vi "FT10_Semi-Auto Tester.vi"(7 "Read/ Write":T8, 8 "Error In":errorcluster, 10 "Semi-Auto Cluster in":T1[](array[typedef]), 11 "Path":path=path "FT10_rev2/Semi-Auto Commands.csv") -> (0 "Error Out":errorcluster, 2 "Semi-Auto Cluster out":T1[](array[typedef]), 3 "Semi-Auto 2-D Array out":T7)   [LabVIEW 2015]
uses:
  LV2024/NI Online Practice/CLD Practice/cld_success_package/Preparation_Materials/CLD 6/CLD 6 CSV file enum.ctl
  Controls/Control_Semi-Auto 2-D Array.ctl
  Controls/Control_Semi-Auto Cluster.ctl
  Controls/Control_Semi-Auto Unitherm Load.ctl
  Controls/Control_Semi-Auto Port.ctl
  Controls/Control_Semi-Auto Mode.ctl
  Controls/Control_Semi-Auto Power Level.ctl
  Controls/Control_Semi-Auto Activation Duration.ctl
  Controls/Control_Semi-Auto 1-D Array.ctl
  <vilib>/Utility/file.llb/Read Delimited Spreadsheet (string).vi
  <vilib>/Utility/file.llb/Write Delimited Spreadsheet (string).vi
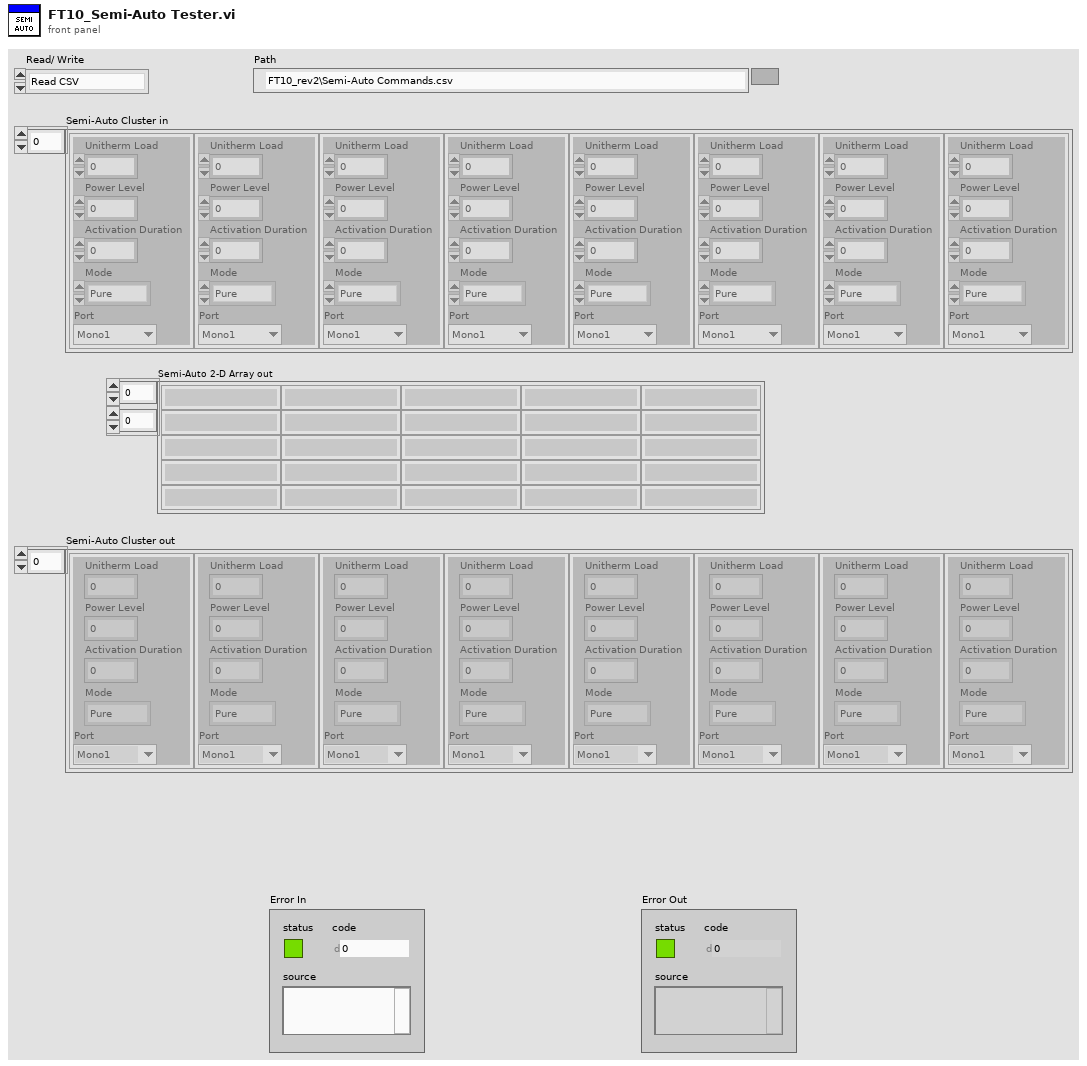
[diagram p1: front panel]
types:
  T1 = typedef "Control_Semi-Auto Cluster.ctl" = cluster{"Unitherm Load":T2, "Port":T3, "Mode":T4, "Power Level":T5, "Activation Duration":T6}
  T2 = typedef "Control_Semi-Auto Unitherm Load.ctl" = i32
  T3 = typedef "Control_Semi-Auto Port.ctl" = enum16{"Mono1", "Mono2", "Bipolar", "Ligasure", "Error"}
  T4 = typedef "Control_Semi-Auto Mode.ctl" = enum16{"Pure", "Blend", "Spray", "Fulgerate", "Standard", "Macro", "Precision", "Ligasure", "Error"}
  T5 = typedef "Control_Semi-Auto Power Level.ctl" = i32
  T6 = typedef "Control_Semi-Auto Activation Duration.ctl" = i32
  T7 = typedef "Control_Semi-Auto 2-D Array.ctl" = string[][]
  T8 = typedef "CLD 6 CSV file enum.ctl" = enum16{"Read CSV", "Write CSV"}
  T9 = typedef "Control_Semi-Auto 1-D Array.ctl" = string[]
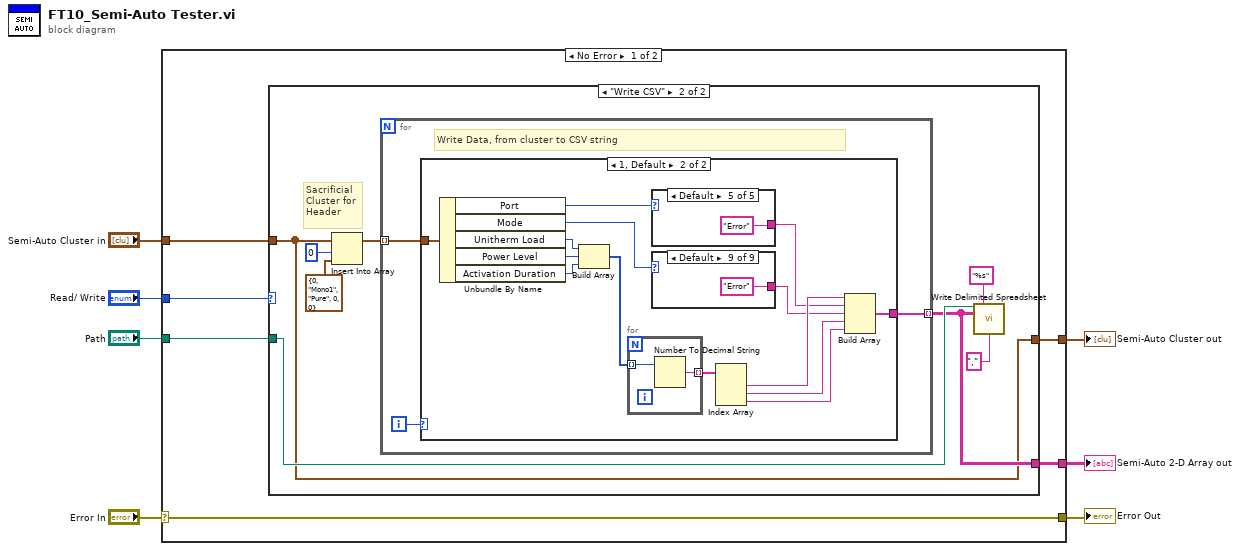
[diagram p0: block diagram]
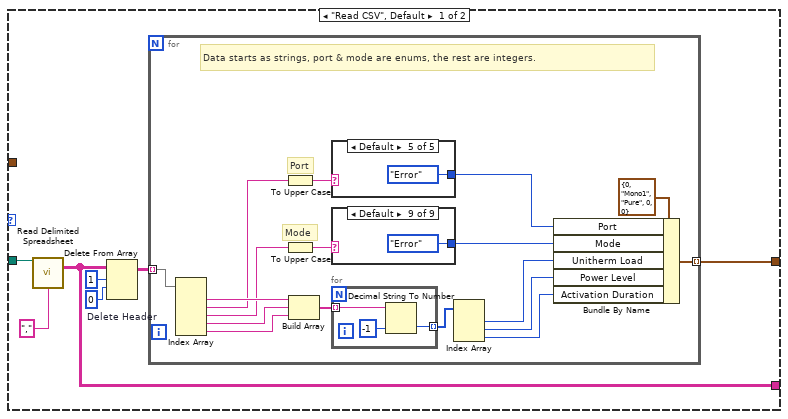
[diagram p2: hidden frame]
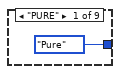
[diagram p3: hidden frame]
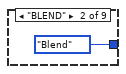
[diagram p4: hidden frame]
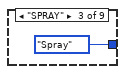
[diagram p5: hidden frame]
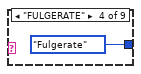
[diagram p6: hidden frame]
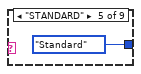
[diagram p7: hidden frame]
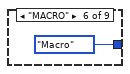
[diagram p8: hidden frame]
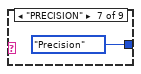
[diagram p9: hidden frame]
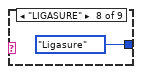
[diagram p10: hidden frame]
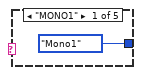
[diagram p11: hidden frame]
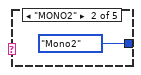
[diagram p12: hidden frame]
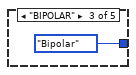
[diagram p13: hidden frame]
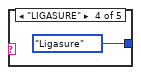
[diagram p14: hidden frame]
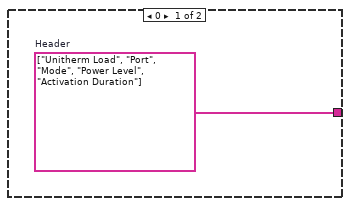
[diagram p15: hidden frame]
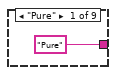
[diagram p16: hidden frame]
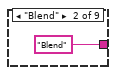
[diagram p17: hidden frame]
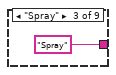
[diagram p18: hidden frame]
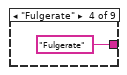
[diagram p19: hidden frame]
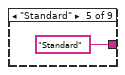
[diagram p20: hidden frame]
diagram:
  n1 = case shown="No Error" "Error In" {
    selector: "Error In" -> [w10 w99]
    tunnel: [w13 T1[] [] ("Semi-Auto Cluster in")] -> w2
    tunnel: "Path" -> [w8 _]
    tunnel: "Read/ Write" -> [w12 _]
    tunnel: "Semi-Auto Cluster in" -> [w11 _]
    tunnel: [w10 w99] -> w4
    tunnel: [w9 string[][] [] ("all rows")] -> w1
    frame No Error {
      n2 = case shown="\"Write CSV\"" w12 {
        tunnel: w8 -> [w19 w61]
        tunnel: [w20 w58] -> w13
        tunnel: w11 -> [_ w58]
        tunnel: [w17 w59] -> w9
        frame "Read CSV", Default {
          n3 = call-poly <vilib>:"Read Delimited Spreadsheet.vi"("file path (dialog if empty)"=w19, "delimiter (\\t)"="," ("delimiter (\\t)")) -> ("all rows"=w17:string[][])  [unwired: 8 in, 5 out]
          n4 = Delete From Array "Delete Header"(array=w17, length=1, index (row)=0) -> (array with subset deleted=w16:string[][])  [unwired: 1 in, 1 out]
          n5 = for {
            tunnel: w16 -> [w36] mode=indexing
            tunnel: [w37] -> w20 mode=indexing
            # "Mode"
            # "Port"
            # "Data starts as strings, port & mode are enums, the rest are integers."
            n6 = Index Array "Index Array"(array=w36) -> (element #1=w35:string, element #2=w31:string, element #3=w30:string, element #4=w34:string, element #5=w33:string)  [unwired: 5 in]
            n7 = To Upper Case(1:w31) -> (0:w24:string)
            n8 = To Upper Case(1:w30) -> (0:w25:string)
            n9 = Build Array(w35, w34, w33) -> (w29:string[])
            n10 = case shown="Default" w24 {
              tunnel: [Control_Semi-Auto_Port."Mono1" ("Port") Control_Semi-Auto_Port."Mono2" ("Port") Control_Semi-Auto_Port."Bipolar" ("Port") Control_Semi-Auto_Port."Ligasure" ("Port") Control_Semi-Auto_Port."Error" ("Port")] -> w22
              frame "MONO1" {
              }
              frame "MONO2" {
              }
              frame "BIPOLAR" {
              }
              frame "LIGASURE" {
              }
              frame Default {
              }
            }
            n11 = case shown="Default" w25 {
              tunnel: [Control_Semi-Auto_Mode."Pure" ("Mode") Control_Semi-Auto_Mode."Blend" ("Mode") Control_Semi-Auto_Mode."Spray" ("Mode") Control_Semi-Auto_Mode."Fulgerate" ("Mode") Control_Semi-Auto_Mode."Standard" ("Mode") Control_Semi-Auto_Mode."Macro" ("Mode") Control_Semi-Auto_Mode."Precision" ("Mode") Control_Semi-Auto_Mode."Ligasure" ("Mode") Control_Semi-Auto_Mode."Error" ("Mode")] -> w21
              frame "PURE" {
              }
              frame "BLEND" {
              }
              frame "SPRAY" {
              }
              frame "FULGERATE" {
              }
              frame "STANDARD" {
              }
              frame "MACRO" {
              }
              frame "PRECISION" {
              }
              frame "LIGASURE" {
              }
              frame Default {
              }
            }
            n12 = for {
              tunnel: w29 -> [w54] mode=indexing
              tunnel: [w53] -> w28 mode=indexing
              n13 = Decimal String To Number(string=w54, default (0L)=-1 ("default (0 I32)")) -> (number=w53:i32)  [unwired: 1 in, 1 out]
            }
            n14 = Index Array "Index Array"(array=w28) -> (element #1=w23:i32, element #2=w27:i32, element #3=w26:i32)  [unwired: 3 in]
            n15 = Bundle By Name(cluster=T1 {"Unitherm Load"=0, "Port"=enum."Mono1", "Mode"=enum."Pure", "Power Level"=0, "Activation Duration"=0}, "Port"=w22, "Mode"=w21, "Unitherm Load"=w23, "Power Level"=w27, "Activation Duration"=w26) -> (w37:T1)
          }
        }
        frame "Write CSV" {
          # "Sacrificial\nCluster for\nHeader"
          n16 = Insert Into Array(array=w58, index=0, new element=T1 {"Unitherm Load"=0, "Port"=enum."Mono1", "Mode"=enum."Pure", "Power Level"=0, "Activation Duration"=0}) -> (w55:T1[])
          n17 = for {
            tunnel: w55 -> [w65] mode=indexing
            tunnel: [w64] -> w59 mode=indexing
            i -> [w63]
            # "Write Data, from cluster to CSV string"
            n18 = case shown="1, Default" w63 {
              tunnel: w65 -> [_ w80]
              tunnel: [w66 w71] -> w64
              frame 0 {
                w66 = T9 ["Unitherm Load", "Port", "Mode", "Power Level", "Activation Duration"]  # Header
              }
              frame 1, Default {
                n19 = Unbundle By Name(w80) -> ("Port"=w70:T3, "Mode"=w69:T4, "Unitherm Load"=w77:T2, "Power Level"=w78:T5, "Activation Duration"=w79:T6)
                n20 = Build Array(w77, w78, w79) -> (w76:T6[])
                n21 = for {
                  tunnel: w76 -> [w96] mode=indexing
                  tunnel: [w95] -> w75 mode=indexing
                  n22 = Number To Decimal String(number=w96) -> (decimal integer string=w95:string)  [unwired: 1 in]
                }
                n23 = case shown="Default" w70 {
                  tunnel: ["Mono1" "Mono2" "Bipolar" "Ligasure" "Error"] -> w67
                  frame "Mono1" {
                  }
                  frame "Mono2" {
                  }
                  frame "Bipolar" {
                  }
                  frame "Ligasure" {
                  }
                  frame Default {
                  }
                }
                n24 = case shown="Default" w69 {
                  tunnel: ["Pure" "Blend" "Spray" "Fulgerate" "Standard" "Macro" "Precision" "Ligasure" "Error"] -> w68
                  frame "Pure" {
                  }
                  frame "Blend" {
                  }
                  frame "Spray" {
                  }
                  frame "Fulgerate" {
                  }
                  frame "Standard" {
                  }
                  frame "Macro" {
                  }
                  frame "Precision" {
                  }
                  frame "Ligasure" {
                  }
                  frame Default {
                  }
                }
                n25 = Index Array(array=w75) -> (element #1=w74:string, element #2=w73:string, element #3=w72:string)  [unwired: 3 in]
                n26 = Build Array(w74, w67, w68, w73, w72) -> (w71:string[])
              }
            }
          }
          n27 = call-poly <vilib>:"Write Delimited Spreadsheet.vi"("file path (dialog if empty)"=w61, "format (%s)"="%s", "2D data"=w59, "delimiter (\\t)"="," ("delimiter (\\t)")) -> ()  [unwired: 10 in, 2 out]
        }
      }
    }
    frame Error {
    }
  }
  "Error Out" <- w4
  "Semi-Auto 2-D Array out" <- w1
  "Semi-Auto Cluster out" <- w2
